vi "Write program file.vi"(8 "error in":errorcluster, 10 "Program in":T1[](array[typedef]), 11 "selected path":path) -> (0 "error out":errorcluster)   [LabVIEW 2014]
uses:
  Teszt.ctl
  Command.ctl
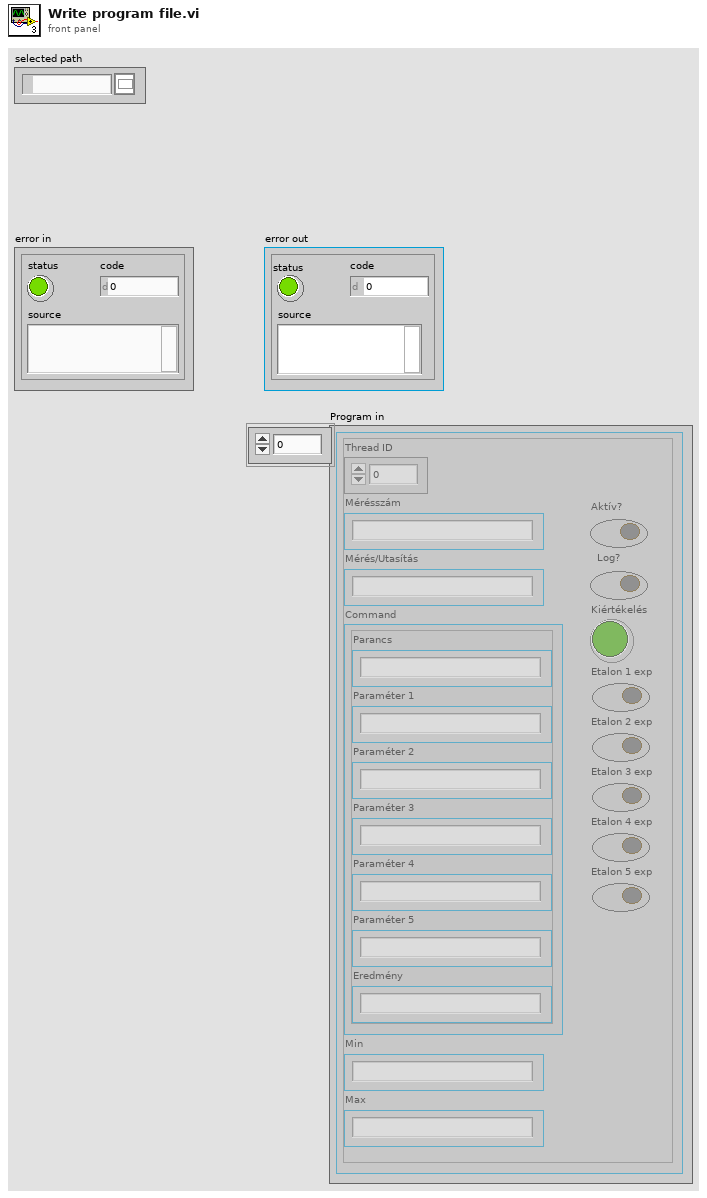
[diagram p1: front panel]
types:
  T1 = typedef "Teszt.ctl" = cluster{"Thread ID":dbl, "Mérésszám":string, "Mérés/Utasítás":string, "Command":T2, "Min":string, "Max":string, "Aktív?":bool, "Log?":bool, "Kiértékelés":bool, "Etalon 1 exp":bool, "Etalon 2 exp":bool, "Etalon 3 exp":bool, "Etalon 4 exp":bool, "Etalon 5 exp":bool}
  T2 = typedef "Command.ctl" = cluster{"Parancs":string, "Paraméter 1":string, "Paraméter 2":string, "Paraméter 3":string, "Paraméter 4":string, "Paraméter 5":string, "Eredmény":string}
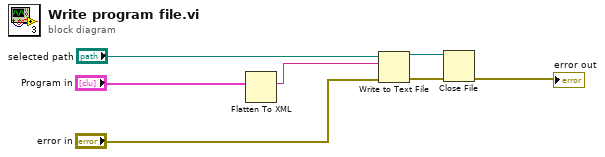
[diagram p0: block diagram]
diagram:
  n1 = Flatten To XML(anything="Program in") -> (xml string=w6:string)
  n2 = Write to Text File(file (use dialog)="selected path", text=w6, error in="error in") -> (refnum out=w3:refnum<file>, error out=w2:errorcluster)  [unwired: 1 in, 1 out]
  n3 = Close File(refnum=w3, error in=w2) -> (error out=→"error out":errorcluster)  [unwired: 1 out]
